vi "BGProcess_DataHandler.vi"(8 "error in (no error)":errorcluster) -> (0 "error out":errorcluster)   [LabVIEW 2012]
uses:
  Controls/Global Stop States.ctl
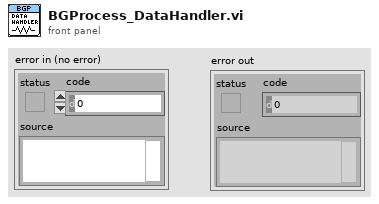
[diagram p1: front panel]
types:
  T1 = typedef "Global Stop States.ctl" = enum16{"STOP", "STATUS", "INIT"}
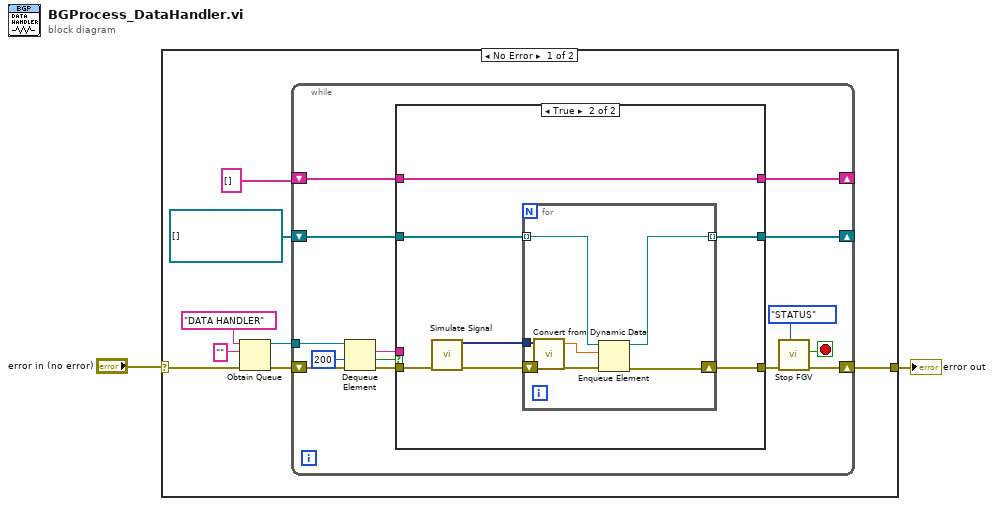
[diagram p0: block diagram]
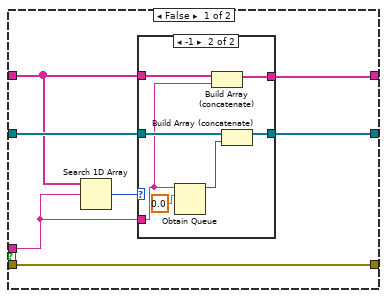
[diagram p2: hidden frame]
diagram:
  n1 = case shown="No Error" "error in (no error)" {
    selector: "error in (no error)" -> [w9 w54]
    tunnel: [w10 w54] -> w2
    frame No Error {
      n2 = Obtain Queue(name (unnamed)="DATA HANDLER", element data type="", error in (no error)=w9) -> (queue out=w7:refnum<queue>, error out=w8:errorcluster)  [unwired: 2 in, 1 out]
      n3 = while {
        shift-right: [w14] -> w10
        shift-left: w8 -> [w24]
        tunnel: w7 -> [w20]
        shift-right: [w17] -> _
        shift-left: refnum<queue>[] [] -> [w18]
        shift-right: [w15] -> _
        shift-left: string[] [] -> [w16]
        stop <- w12 stop-if-true
        n4 = Dequeue Element(queue=w20, timeout in ms (-1)=200, error in (no error)=w24) -> (element=w19:string, timed out?=w22:bool, error out=w23:errorcluster)  [unwired: 1 out]
        n5 = case shown="True" w22 {
          tunnel: w23 -> [w28 w47]
          tunnel: [w28 w41] -> w13
          tunnel: w19 -> [w27 _]
          tunnel: w18 -> [w30 w45]
          tunnel: [w29 w44] -> w17
          tunnel: w16 -> [w26 w43]
          tunnel: [w25 w43] -> w15
          frame False {
            n6 = Search 1D Array(1D array=w26, element=w27) -> (index of element=w31:i32)  [unwired: 1 in]
            n7 = case shown="-1" w31 {
              tunnel: w30 -> [w33 w40]
              tunnel: w27 -> [_ w36]
              tunnel: [w33 w39] -> w29
              tunnel: w26 -> [w32 w37]
              tunnel: [w32 w35] -> w25
              frame Default {
              }
              frame -1 {
                n8 = Obtain Queue(name (unnamed)=w36, element data type=0.0) -> (queue out=w38:refnum<queue>)  [unwired: 3 in, 2 out]
                n9 = Build Array (concatenate)(w37, w36) -> (w35:string[])
                n10 = Build Array (concatenate)(w40, w38) -> (w39:refnum<queue>[])
              }
            }
          }
          frame True {
            n11 = call "Simulate Signal"("error in (no error)"=w47) -> ("Sine"=w42:dynamicdata, "error out"=w46:errorcluster)  [unwired: 13 in]
            n12 = for {
              shift-right: [w50] -> w41
              shift-left: w46 -> [w53]
              tunnel: w45 -> [w49] mode=indexing
              tunnel: [w48] -> w44 mode=indexing
              tunnel: w42 -> [w52]
              n13 = call "Convert from Dynamic Data"("Dynamic Data Type"=w52) -> ("Scalar"=w51:dbl)  [unwired: 3 in]
              n14 = Enqueue Element(queue=w49, element=w51, error in (no error)=w53) -> (queue out=w48:refnum<queue>, error out=w50:errorcluster)  [unwired: 1 in, 1 out]
            }
          }
        }
        n15 = call "Stop FGV.vi"("Operation In"=Global_Stop_States."STATUS", "error in"=w13) -> ("error out"=w14:errorcluster, "Stop?"=w12:bool)  [unwired: 8 in]
      }
    }
    frame Error {
    }
  }
  "error out" <- w2
